vi "Configure Trigger Characteristics (RF Burst).vi"(6 "Trigger Level Value (1 dB)":dbl=1.0, 7 "Enable Narrow Pulse Discriminator (T: Enable)":bool=TRUE, 8 "error in (no error)":errorcluster, 9 "Trigger Level Type (0: Absolute)":u16(ring) items=["Absolute", "Relative"], 10 "Enable RF Burst Selectivity (T: Enable)":bool=TRUE, 11 "VISA resource name":refnum<visa-resource-name>) -> (0 "error out":errorcluster, 3 "VISA resource name out":refnum<visa-resource-name>)   [LabVIEW 2014, in "Agilent ESA PSA Series.lvlib"]
doc: "Configures the trigger settings for RF Burst.It is applicable when the trigger source is set to RF trigger and Option B7E is installed."
uses:
  Agilent ESA PSA Series.lvlib
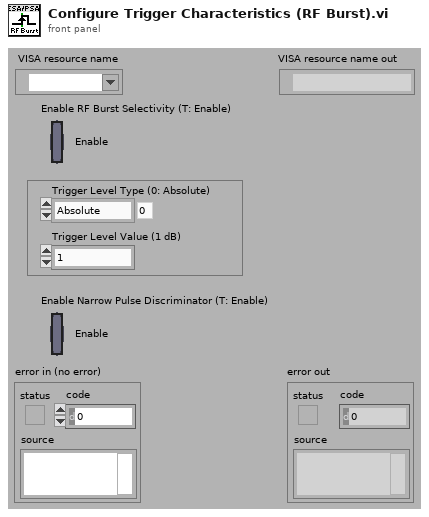
[diagram p1: front panel]
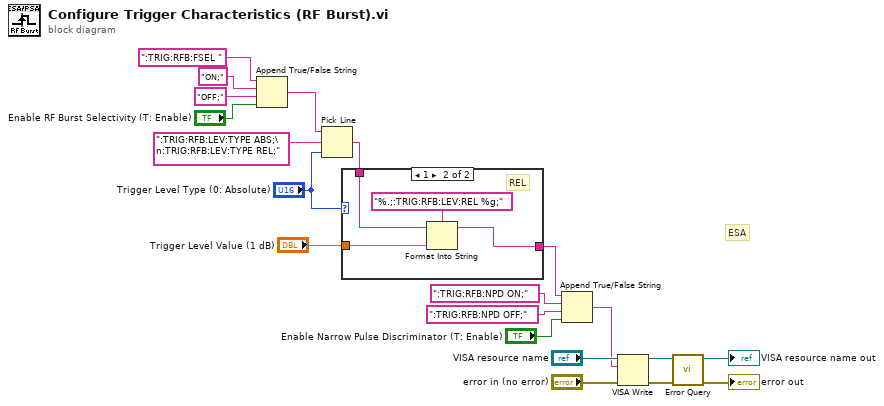
[diagram p0: block diagram]
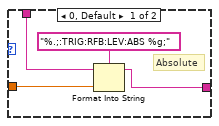
[diagram p2: hidden frame]
diagram:
  # "ESA"
  n1 = Append True/False String(1:"Enable RF Burst Selectivity (T: Enable)", 2:"OFF;" ("string (\"\")"), 3:"ON;" ("string (\"\")"), 4:":TRIG:RFB:FSEL " ("string (\"\")")) -> (0:w2:string)
  n2 = Pick Line(string ("")=w2, multi-line string=":TRIG:RFB:LEV:TYPE ABS;\n:TRIG:RFB:LEV:TYPE REL;", line index="Trigger Level Type (0: Absolute)") -> (output string=w8:string)
  n3 = case shown="1" "Trigger Level Type (0: Absolute)" {
    tunnel: "Trigger Level Value (1 dB)" -> [w23 w25]
    tunnel: w8 -> [w22 w27]
    tunnel: [w21 w26] -> w5
    frame 0, Default {
      # "Absolute"
      n4 = Format Into String(format string="%.;:TRIG:RFB:LEV:ABS %g;", initial string=w22, w23) -> (resulting string=w21:string)  [unwired: 1 in, 1 out]
    }
    frame 1 {
      # "REL"
      n5 = Format Into String(format string="%.;:TRIG:RFB:LEV:REL %g;", initial string=w27, w25) -> (resulting string=w26:string)  [unwired: 1 in, 1 out]
    }
  }
  n6 = Append True/False String(1:"Enable Narrow Pulse Discriminator (T: Enable)", 2:":TRIG:RFB:NPD OFF;" ("true string"), 3:":TRIG:RFB:NPD ON;" ("true string"), 4:w5) -> (0:w1:string)
  n7 = VISA Write(VISA resource name="VISA resource name", write buffer=w1, error in (no error)="error in (no error)") -> (VISA resource name out=w18:refnum<visa-resource-name>, error out=w16:errorcluster)  [unwired: 1 out]
  n8 = call "Error Query.vi"("error in (no error)"=w16, "VISA resource name"=w18) -> ("error out"=→"error out":errorcluster, "VISA resource name out"=→"VISA resource name out":refnum<visa-resource-name>)  [unwired: 6 in, 2 out]
